vi "escribeListaDePruebas.vi"(8 "error in (no error)":errorcluster, 11 "Equipo in":refnum<class "Equipo.lvclass">) -> (0 "error out":errorcluster, 3 "Equipo out":refnum<class "Equipo.lvclass">)   [LabVIEW 2019, in "Equipo.lvclass"]
uses:
  Equipo.lvclass
  Equipo.lvclass/Equipo.ctl
  Base de Datos/Base de Datos.lvclass
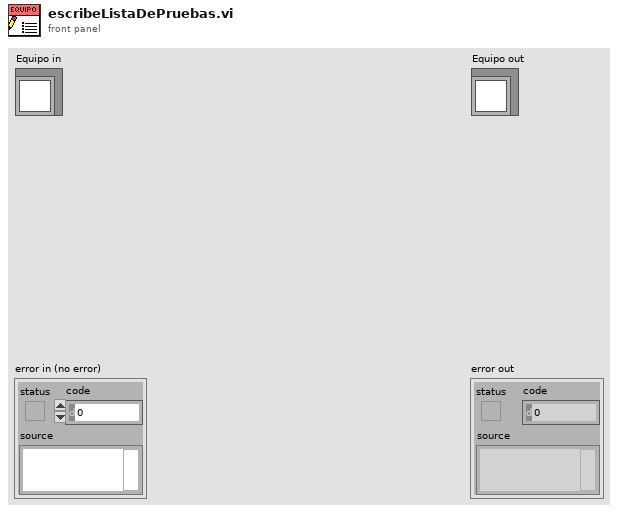
[diagram p1: front panel]
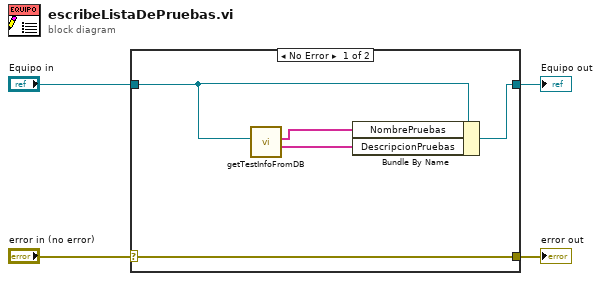
[diagram p0: block diagram]
diagram:
  n1 = case shown="No Error" "error in (no error)" {
    selector: "error in (no error)" -> [w9 w10]
    tunnel: [w9 w10] -> w3
    tunnel: [w8 w11] -> w1
    tunnel: "Equipo in" -> [w7 w11]
    frame No Error {
      n2 = call "getTestInfoFromDB.vi"("Equipo.lvclass"=w7) -> ("DescripcionPruebas"=w6:string[], "NombrePruebas"=w5:string[])  [unwired: 7 in, 2 out]
      n3 = Bundle By Name(cluster=w7, "NombrePruebas"=w5, "DescripcionPruebas"=w6) -> (w8:refnum<class "Equipo.lvclass">)
    }
    frame Error {
    }
  }
  "error out" <- w3
  "Equipo out" <- w1
